vi "Load SVG From Memory (Core).vi"(8 "error in (no error)":errorcluster, 10 "Scale (1)":dbl=1.0, 11 "Encoded Image":u8[](array[numeric])) -> (0 "error out":errorcluster, 2 "Extended Image":T1)   [LabVIEW 2020, in "G-Image.lvlib"]
doc: "Load an image file from disk."
uses:
  G-Image.lvlib
  <vilib>/picture/picture.llb/imagedata.ctl
  Private/Extended Image.ctl
  lib/g_image_32.dll
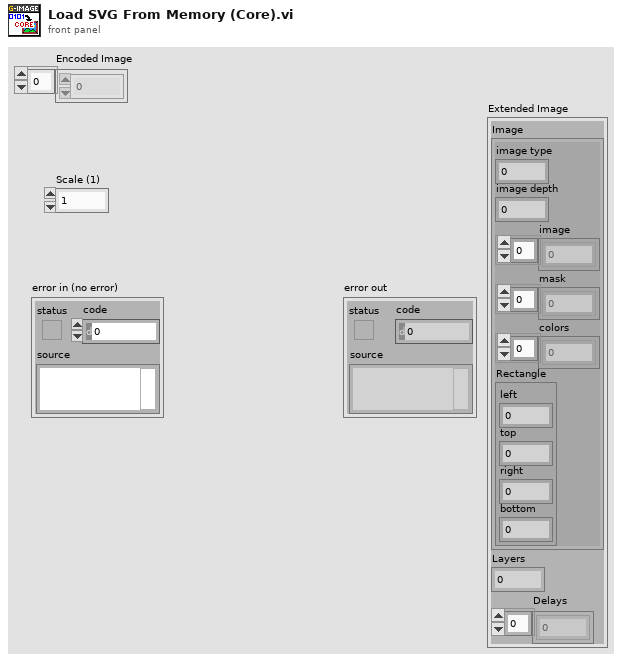
[diagram p1: front panel]
types:
  T1 = typedef "G-Image.lvlib/Extended Image.ctl" = cluster{"Image":T2, "Layers":i32, "Delays":i32[]}
  T2 = typedef "imagedata.ctl" = cluster{"image type":i32, "image depth":i32, "image":u8[], "mask":u8[], "colors":u32[], "Rectangle":cluster{"left":i16, "top":i16, "right":i16, "bottom":i16}}
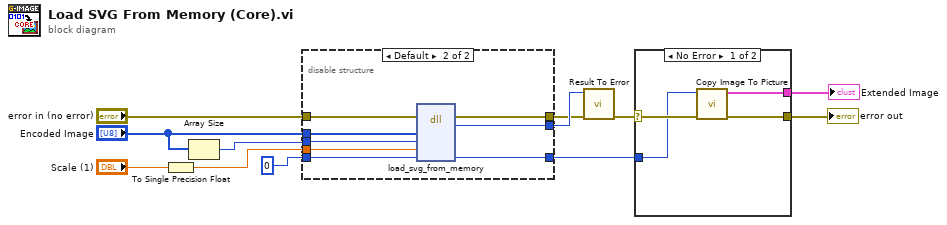
[diagram p0: block diagram]
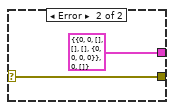
[diagram p2: hidden frame]
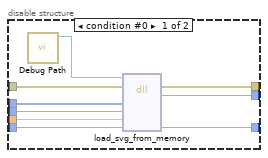
[diagram p3: hidden frame]
diagram:
  n1 = To Single Precision Float(number="Scale (1)") -> (single precision float=w3:sgl)
  n2 = Array Size(array="Encoded Image") -> (size(s)=w1:i32)
  n3 = disable-structure shown="Default" {
    disable-tunnel: [w20 w29] -> w9
    disable-tunnel: "error in (no error)" -> [w19 w28]
    disable-tunnel: "Encoded Image" -> [w18 w27]
    disable-tunnel: [w17 w26] -> w10
    disable-tunnel: [w16 w24] -> w6
    disable-tunnel: i64 0 ("count") -> [w15 w25]
    disable-tunnel: w3 -> [w14 w23]
    disable-tunnel: w1 -> [w13 w22]
    frame condition #0 {
      n4 = call "Debug Path.vi"() -> ("Debug Path"=w21:path)  [unwired: 11 in]
      n5 = dll-call lib="?" fn="load_svg_from_memory"(path in=w21, error in=w19, "encoded_image"=w18, "encoded_image_count"=w13, "scale"=w14, "image_out"=w15) -> (error out=w20:errorcluster, "result"=w17:i32, "image_out"=w16:i64)  [unwired: 4 in, 1 out]
    }
    frame condition #1 (active) {
      n6 = dll-call lib="C:/github/dataflowg/g-image/src/LabVIEW/G-Image/lib/g_image_*.*" fn="load_svg_from_memory"(error in=w28, "encoded_image"=w27, "encoded_image_count"=w22, "scale"=w23, "image_out"=w25) -> (error out=w29:errorcluster, "result"=w26:i32, "image_out"=w24:i64)  [unwired: 5 in, 1 out]
    }
  }
  n7 = call "Result To Error.vi"("error in (no error)"=w9, "Result Code"=w10) -> ("error out"=w8:errorcluster)  [unwired: 9 in]
  n8 = case shown="No Error" w8 {
    selector: w8 -> [w33 w35]
    tunnel: [w31 w35] -> w12
    tunnel: w6 -> [w32 _]
    tunnel: [w30 T1 {"Image"={"image type"=0, "image depth"=0, "image"=[], "mask"=[], "colors"=[], "Rectangle"={"left"=0, "top"=0, "right"=0, "bottom"=0}}, "Layers"=0, "Delays"=[]} ("Image")] -> w5
    frame No Error {
      n9 = call "Copy Image To Picture.vi"("error in (no error)"=w33, "image_ptr"=w32) -> ("error out"=w31:errorcluster, "Extended Image"=w30:T1)  [unwired: 8 in]
    }
    frame Error {
    }
  }
  "error out" <- w12
  "Extended Image" <- w5
